vi "Check Step Action Visibility.vi"(11 "Step Settings in":T1) -> (2 "Actions visible":bool, 3 "Step Settings out":T1)   [LabVIEW 2024, in "Output Sequencer.lvlib" / "Settings UI.lvclass"]
uses:
  Settings UI.lvclass
  Types/Step Settings.ctl
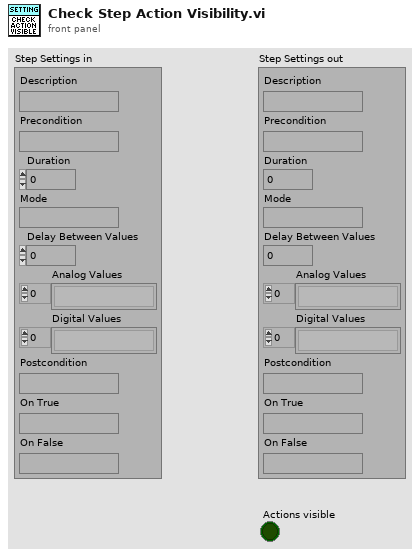
[diagram p1: front panel]
types:
  T1 = typedef "Output Sequencer.lvlib/Settings UI.lvclass/Step Settings.ctl" = cluster{"Description":string, "Precondition":string, "Duration":dbl, "Mode":string, "Delay Between Values":dbl, "Analog Values":string[], "Digital Values":string[], "Postcondition":string, "On True":string, "On False":string}
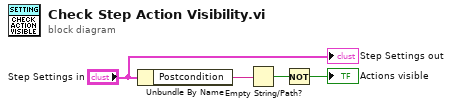
[diagram p0: block diagram]
diagram:
  n1 = Unbundle By Name("Step Settings in") -> ("Postcondition"=w4:string)
  n2 = Empty String/Path?(string/path=w4) -> (empty?=w3:bool)
  n3 = Not(x=w3) -> (.not. x?=→"Actions visible":bool)
  "Step Settings out" <- "Step Settings in"
